vi "UHR-Fleezers Control (host) - 10.8.vi"() -> ()   [LabVIEW 2013] (continued)
            n877 = local read "Pump write delay (ms)"() -> (w1433:dbl)
            n878 = flat-sequence {
              tunnel: w1432 -> [w1446]
              tunnel: w1433 -> [w1442]
              tunnel: w1431 -> [_]
              tunnel: w1433 -> [w1448]
              tunnel: w1432 -> [w1449]
              frame #0 {
                n879 = local read "All Pump Parameters"() -> (w1441:T5)
                n880 = Multiply(x=60.0, y="Flush Center Ch Rate (ul/m)") -> (x*y=w1438:dbl)
                n881 = Unbundle By Name(w1441) -> ("Pump 2"=w1447:T35)
                n882 = call "Set pump parameters.vi"("Pump write delay (ms)"=w1442, "Volume (uL)"="Flush Center Ch Volume (uL)", "Rate (uL/h)"=w1438, "Units"=3.0, "Pump #"=2.0, "Pump Parameters In"=w1447, "VISA resource name"=w1446) -> ("Pump Parameters Out"=w1440:T35)  [unwired: 3 in]
                n883 = Bundle By Name(cluster=w1441, "Pump 2"=w1440) -> (w1439:T5)
                n884 = local write "All Pump Parameters"(w1439) -> ()
                n885 = Add(x="Flush Center Ch Volume (uL)", y="Total Volume\nFlushed (uL)") -> (x+y=w1435:dbl)
                n886 = local write "Total Volume\nFlushed (uL)"(w1435) -> ()
              }
              frame #1 {
                n887 = Wait (ms)(milliseconds to wait=w1448) -> ()  [unwired: 1 out]
              }
              frame #2 {
                n888 = call "Write to pump.vi"("string"="start", "VISA resource name"=w1449) -> ()  [unwired: 1 out]
              }
            }
            n889 = local read "Chemyx Syringe Pump Serial Port"() -> (w1432:refnum<visa-resource-name>)
          }
          frame Enabled {
            n890 = call "hamilton_controller.vi"("Open?"=w1451, "valve"=enum16{"A", "B", "C", "D", "ALL"}."B", "action"=T21."MOVE VALVE") -> ()  [unwired: 8 in, 1 out]
          }
        }
      }
      event "Sample Channel Flow": Value Change {
        n891 = event-data() -> ()  [unwired: 7 out]
        n892 = call "hamilton_controller.vi"("Open?"="Sample Channel Flow", "valve"=enum16{"A", "B", "C", "D", "ALL"}."C", "action"=T21."MOVE VALVE") -> ()  [unwired: 8 in, 1 out]
      }
      event "Flip Green Filter": Value Change {
        n893 = event-data() -> ()  [unwired: 7 out]
        n894 = Not(x="Flip Green Filter") -> (.not. x?=w1457:bool)
        n895 = local write "Flip Green Filter"(w1457) -> ()
        n896 = flat-sequence {
          tunnel: w1465 -> [w1470]
          tunnel: w1464 -> [w1469]
          tunnel: [w1467] -> w1462
          tunnel: [w1466] -> w1461
          tunnel: [w1472] -> w1460
          tunnel: w1462 -> [w1472]
          tunnel: [w1471] -> w1459
          tunnel: w1461 -> [w1471]
          tunnel: w1460 -> [w1476]
          tunnel: w1459 -> [w1475]
          tunnel: [w1474] -> w1463
          frame #0 {
            n897 = xnode "Read/Write Control"("FPGA VI Reference In"=w1470, "error in"=w1469, "Green Filter Flipper"=TRUE) -> ("FPGA VI Reference Out"=w1467:T19, "error out"=w1466:errorcluster)
          }
          frame #1 {
            n898 = Wait (ms)(milliseconds to wait=u32 100) -> ()  [unwired: 1 out]
          }
          frame #2 {
            n899 = xnode "Read/Write Control"("FPGA VI Reference In"=w1476, "error in"=w1475, "Green Filter Flipper"=FALSE) -> ("error out"=w1474:errorcluster)  [unwired: 1 out]
          }
        }
      }
      event "Pump 1 contents", "Pump 3 contents": Value Change {
        n900 = event-data() -> ()  [unwired: 7 out]
        n901 = local read "Pump 1 contents"() -> (→"Pump 1 cont disp":string)
        n902 = local read "Pump 3 contents"() -> (→"Pump 3 cont disp":string)
      }
      event "Reset Trap Pos. FB": Value Change {
        n903 = event-data() -> ()  [unwired: 7 out]
        n904 = xnode "Read/Write Control"("FPGA VI Reference In"=w1482, "error in"=w1481, "Trap Pos. FB Reset"="Reset Trap Pos. FB") -> ()  [unwired: 2 out]
      }
      event "Trap Pos. FB ON": Value Change {
        n905 = event-data() -> ()  [unwired: 7 out]
        n906 = xnode "Read/Write Control"("FPGA VI Reference In"=w1485, "error in"=w1484, "Force feedback"="Trap Pos. FB ON") -> ()  [unwired: 2 out]
      }
      event "Trap Pos. FB Range", "Trap Pos. FB Gains", "Trap Pos. FB Mult Factor", "Trap Pos. FB Offset Factor", "Trap Pos FB Negate Action", "Trap Pos FB Monitor\nT1 or T2": Value Change {
        n907 = event-data() -> ()  [unwired: 7 out]
        n908 = xnode "Read/Write Control"("FPGA VI Reference In"=w1494, "error in"=w1493, "Trap Pos. FB Range"="Trap Pos. FB Range", "Trap Pos. FB Gains"="Trap Pos. FB Gains", "Trap Pos. FB Mult Factor"="Trap Pos. FB Mult Factor", "Trap Pos. FB Offset Factor"="Trap Pos. FB Offset Factor", "Trap Pos FB Negate Action"="Trap Pos FB Negate Action", "Trap Pos FB Monitor T1 or T2"="Trap Pos FB Monitor\nT1 or T2", "AI1 X Scale"="Trap Pos. AI1 X Pre-scale") -> ()  [unwired: 2 out]
      }
      event "Trap Pos FB SP": Value Change {
        n909 = event-data() -> ()  [unwired: 7 out]
        n910 = xnode "Read/Write Control"("FPGA VI Reference In"=w1497, "error in"=w1496, "Trap Pos. FB SP"="Trap Pos FB SP") -> ()  [unwired: 2 out]
      }
      event "Set SP to Reading": Value Change {
        n911 = event-data() -> ()  [unwired: 7 out]
        n912 = local read "Trap Pos FB Monitor\nT1 or T2"() -> (w1505:bool)
        n913 = local read "Trap X AI1 (DMA)"() -> (w1508:T13)
        n914 = local read "Trap X (AI1)"() -> (w1511:T10)
        n915 = Unbundle By Name(w1511) -> ("Trap 1"=w1510:fxp<+/-,16,1>, "Trap 2"=w1509:fxp<+/-,16,1>)
        n916 = Unbundle By Name(w1508) -> ("Set 1"=w1507:fxp<+/-,16,1>, "Set 2"=w1506:fxp<+/-,16,1>)
        n917 = Select(t=w1510, s=w1505, f=w1509) -> (s? t:f=w1504:fxp<+/-,16,1>)
        n918 = Select(t=w1507, s=w1505, f=w1506) -> (s? t:f=w1503:fxp<+/-,16,1>)
        n919 = Not(x="Set SP Using...") -> (.not. x?=w1498:bool)
        n920 = Select(t=w1504, s=w1498, f=w1503) -> (s? t:f=w1499:fxp<+/-,16,1>)
        n921 = xnode "Read/Write Control"("FPGA VI Reference In"=w1501, "error in"=w1500, "Trap Pos. FB SP"=w1499) -> ()  [unwired: 2 out]
        n922 = local write "Trap Pos FB SP"(w1499) -> ()
      }
      event "Trap Pos. FB Out Scale 2^n": Value Change {
        n923 = event-data() -> ()  [unwired: 7 out]
        n924 = Scale By Power Of 2(n="Trap Pos. FB Out Scale 2^n", x=ext 1.0) -> (x*2^n=w1513:ext)
        n925 = property on="Trap Pos. FB Mult Factor" class="DigNum (strict)"("Val(Sgnl)"=w1513) -> ()  [unwired: 2 in, 2 out]
      }
      event "Trap Pos FB Int Count": Value Change {
        n926 = event-data() -> ()  [unwired: 7 out]
        n927 = xnode "Read/Write Control"("FPGA VI Reference In"=w1518, "error in"=w1517, "Trap Pos FB Int Count"="Trap Pos FB Int Count") -> ()  [unwired: 2 out]
      }
    }
    "error out 2" <- w637
    n928 = node-c288() -> ()  [unwired: 1 in, 1 out]
  }
  n929 = timed-loop "Run Scripts, including: stage motion" {
    timing: w68 -> [_]
    timing-out: [_] -> w67
    tunnel: w16 -> [_]
    stop <- w1520 stop-if-true
    n930 = node-c288() -> ()  [unwired: 1 in, 1 out]
    n931 = event shown="[10] \"Move to Position 1\", \"Move to Position 2\", \"Move to Position 3\", \"Move to Position 4\", \"Move to Position 5\", \"Lower Ch. Cap.\": Value Change" {
      selector: _ -> [_ _ _ _ _ _ _ _ _ _ _ _ _ _ _ _ _]
      dyn-events: _ -> [_ _ _ _ _ _ _ _ _ _ _ _ _ _ _ _ _]
      timeout: 50 -> [_ _ _ _ _ _ _ _ _ _ _ _ _ _ _ _ _]
      tunnel: ["Set Position" "Move to Position" "Move Cap. 1 (DNA Top)" _ "Move Cap. 2 (ADig Bot)" _ "Cal/Data Acq. Spot" "Dump Beads" "Dip for Protein" _ _ "Got ADig bead" "Got DNA bead" "Take Stepping Data" _ "Take Detection Laser\nImage" _] -> _
      tunnel: [_ _ _ _ _ _ _ _ _ _ _ _ _ _ _ _ w1905] -> w1520
      event "Set Position", "Set Position 2", "Set Position 3", "Set Position 4", "Set Position 5", "Set Position 1": Value Change {
        n932 = event-data() -> ()  [unwired: 1 in, 5 out]
        n933 = Build Array("Set Position 1", "Set Position 2", "Set Position 3", "Set Position 4", "Set Position 5") -> (w1539:bool[])
        n934 = Boolean Array To Number(Boolean array=w1539) -> (number=w1538:u32)
        n935 = Logarithm Base 2(1:w1538) -> (0:w1530:dbl)
        n936 = call "CONEX_FUNCTIONAL_GLOBAL.vi"("Command"=T20."GET POS") -> ("Current Position"=w1523:dbl[])  [unwired: 8 in, 2 out]
        n937 = Decrement(x="Position") -> (x-1=w1528:dbl)
        n938 = Greater Or Equal?(x=w1530, y=0.0) -> (x >= y?=w1531:bool)
        n939 = Select(t=w1530, s=w1531, f=w1528) -> (s? t:f=w1527:dbl)
        n940 = Increment(x=w1527) -> (x+1=w1526:dbl)
        n941 = Build Array (concatenate)(w1526, w1523) -> (w1525:dbl[])
        n942 = Replace Array Subset(array="Saved Stage Positions", new element=w1525, index (row)=w1527) -> (w1540:dbl[][])  [unwired: 1 in]
        n943 = local write "Saved Stage Positions"(w1540) -> ()
      }
      event "Move to Position": Value Change {
        n944 = event-data() -> ()  [unwired: 1 in, 5 out]
        n945 = flat-sequence {
          frame #0 {
            n946 = local read "Position"() -> (w1555:dbl)
            n947 = local read "Saved Stage Positions"() -> (w1553:dbl[][])
            n948 = Decrement(x=w1555) -> (x-1=w1552:dbl)
            n949 = Array Subset(array=w1553, index (row)=w1552, length (row)=1 ("length"), index (col)=1 ("index"), length (col)=3 ("length")) -> (w1549:dbl[][])
            n950 = Reshape Array(w1549, 3 ("dimension size")) -> (w1545:dbl[])
            n951 = local write "Stage Moving"(TRUE ("Stage Moving")) -> ()
            n952 = call "CONEX_FUNCTIONAL_GLOBAL.vi"("Axis"=enum16{"X", "Y", "Z", "XY", "XZ", "YZ", "XYZ"}."XYZ", "Position"=w1545, "Command"=T20."ABS MOVE") -> ()  [unwired: 6 in, 3 out]
          }
          frame #1 {
            n953 = call "motor_done_moving.vi"("wait at least (s)"=0.0) -> ()  [unwired: 11 in]
          }
          frame #2 {
            n954 = call <vilib>:"Beep.vi"() -> ()  [unwired: 3 in, 9 out]
            n955 = local write "Stage Moving"(FALSE ("Stage Moving")) -> ()
          }
        }
      }
      event "Move Cap. 1 (DNA Top)": Value Change {
        n956 = event-data() -> ()  [unwired: 1 in, 5 out]
        n957 = local write "Move Cap. 1 (DNA Top)"(FALSE ("Move Cap. 1 (DNA Right)")) -> ()
        n958 = flat-sequence {
          tunnel: ["Cap 1 Samp Flow ON"] -> w1559
          tunnel: w1559 -> [w1578]
          tunnel: [w1578] -> w1558
          tunnel: w1558 -> [w1579]
          frame #0 {
            n959 = local read "Saved Stage Positions"() -> (w1572:dbl[][])
            n960 = Array Subset(array=w1572, index (row)=0 ("index"), length (row)=1 ("length"), index (col)=1 ("index"), length (col)=3 ("length")) -> (w1569:dbl[][])
            n961 = Reshape Array(w1569, 3 ("dimension size")) -> (w1563:dbl[])
            n962 = case "start flow in central channel to wash" shown="True" "Cap 1 Samp Flow ON" {
              frame False {
              }
              frame True {
                n963 = call "hamilton_controller.vi"("Open?"=TRUE, "valve"=enum16{"A", "B", "C", "D", "ALL"}."C", "action"=T21."MOVE VALVE") -> ()  [unwired: 8 in, 1 out]
              }
            }
            n964 = call "CONEX_FUNCTIONAL_GLOBAL.vi"("Axis"=enum16{"X", "Y", "Z", "XY", "XZ", "YZ", "XYZ"}."XYZ", "Position"=w1563, "Command"=T20."ABS MOVE") -> ()  [unwired: 6 in, 3 out]
            n965 = local write "Stage Moving"(TRUE ("Stage Moving")) -> ()
          }
          frame #1 {
            n966 = call "motor_done_moving.vi"("wait at least (s)"=2.0) -> ()  [unwired: 11 in]
          }
          frame #2 {
            n967 = local write "Stage Moving"(FALSE ("Stage Moving")) -> ()
            n968 = case "stop flow" shown="True" w1579 {
              frame False {
              }
              frame True {
                n969 = call "hamilton_controller.vi"("Open?"=FALSE, "valve"=enum16{"A", "B", "C", "D", "ALL"}."C", "action"=T21."MOVE VALVE") -> ()  [unwired: 8 in, 1 out]
              }
            }
            n970 = case shown="True" TRUE {
              tunnel: "Cap 1 T ON" -> [w1588 w1589]
              frame False {
                n971 = property on="Trap 1 (ON/OFF)" class="Bool (strict)"("Val(Sgnl)"=w1588) -> ()  [unwired: 2 in, 2 out]
              }
              frame True {
                n972 = property on="Trap 2 (ON/OFF)" class="Bool (strict)"("Val(Sgnl)"=w1589) -> ()  [unwired: 2 in, 2 out]
              }
            }
            n973 = call <vilib>:"Beep.vi"() -> ()  [unwired: 3 in, 9 out]
            n974 = case shown="True" "Cap 1 Flow ON" {
              frame False {
              }
              frame True {
                n975 = property on="Inject Top" class="Bool (strict)"("Val(Sgnl)"=TRUE ("Value (Signaling)")) -> ()  [unwired: 2 in, 2 out]
              }
            }
          }
        }
      }
      event Timeout {
        n976 = event-data() -> ()  [unwired: 1 in, 2 out]
      }
      event "Move Cap. 2 (ADig Bot)": Value Change {
        n977 = event-data() -> ()  [unwired: 1 in, 5 out]
        n978 = local write "Move Cap. 2 (ADig Bot)"(FALSE ("Move Cap. 2 (ADig Left)")) -> ()
        n979 = flat-sequence {
          tunnel: ["Cap 2 Samp Flow ON"] -> w1591
          tunnel: w1591 -> [w1610]
          tunnel: [w1610] -> w1590
          tunnel: w1590 -> [w1611]
          frame #0 {
            n980 = local read "Saved Stage Positions"() -> (w1604:dbl[][])
            n981 = case shown="True" "Cap 2 Samp Flow ON" {
              frame False {
              }
              frame True {
                n982 = call "hamilton_controller.vi"("Open?"=TRUE, "valve"=enum16{"A", "B", "C", "D", "ALL"}."C", "action"=T21."MOVE VALVE") -> ()  [unwired: 8 in, 1 out]
              }
            }
            n983 = Array Subset(array=w1604, index (row)=1 ("index"), length (row)=1 ("length"), index (col)=1 ("index"), length (col)=3 ("length")) -> (w1601:dbl[][])
            n984 = Reshape Array(w1601, 3 ("dimension size")) -> (w1595:dbl[])
            n985 = local write "Stage Moving"(TRUE ("Stage Moving")) -> ()
            n986 = call "CONEX_FUNCTIONAL_GLOBAL.vi"("Axis"=enum16{"X", "Y", "Z", "XY", "XZ", "YZ", "XYZ"}."XYZ", "Position"=w1595, "Command"=T20."ABS MOVE") -> ()  [unwired: 6 in, 3 out]
          }
          frame #1 {
            n987 = call "motor_done_moving.vi"("wait at least (s)"=2.0) -> ()  [unwired: 11 in]
          }
          frame #2 {
            n988 = local write "Stage Moving"(FALSE ("Stage Moving")) -> ()
            n989 = case shown="True" TRUE {
              tunnel: "Cap 2 T ON" -> [w1620 w1621]
              frame False {
                n990 = property on="Trap 2 (ON/OFF)" class="Bool (strict)"("Val(Sgnl)"=w1620) -> ()  [unwired: 2 in, 2 out]
              }
              frame True {
                n991 = property on="Trap 1 (ON/OFF)" class="Bool (strict)"("Val(Sgnl)"=w1621) -> ()  [unwired: 2 in, 2 out]
              }
            }
            n992 = call <vilib>:"Beep.vi"() -> ()  [unwired: 3 in, 9 out]
            n993 = case shown="True" w1611 {
              frame False {
              }
              frame True {
                n994 = call "hamilton_controller.vi"("Open?"=FALSE, "valve"=enum16{"A", "B", "C", "D", "ALL"}."C", "action"=T21."MOVE VALVE") -> ()  [unwired: 8 in, 1 out]
              }
            }
            n995 = case shown="True" "Cap 2 Flow ON" {
              frame False {
              }
              frame True {
                n996 = property on="Inject Bottom" class="Bool (strict)"("Val(Sgnl)"=TRUE ("Value (Signaling)")) -> ()  [unwired: 2 in, 2 out]
              }
            }
          }
        }
      }
      event "+z", "-z": Value Change {
        n997 = event-data() -> ()  [unwired: 1 in, 5 out]
        n998 = flat-sequence {
          frame #0 {
            w1623 = 0.0 ("element")
            n999 = Divide(x="z nudge increment (um)", y=1000.0) -> (x/y=w1636:dbl)
            n1000 = Boolean To (0,1)(Boolean="+z") -> (0, 1=w1629:i16)
            n1001 = Boolean To (0,1)(Boolean="-z") -> (0, 1=w1630:i16)
            n1002 = Multiply(x=w1629, y=w1636) -> (x*y=w1633:dbl)
            n1003 = Multiply(x=w1630, y=w1636) -> (x*y=w1631:dbl)
            n1004 = Negate(x=w1631) -> (-x=w1632:dbl)
            n1005 = Add(x=w1633, y=w1632) -> (x+y=w1624:dbl)
            n1006 = Build Array(w1623, w1623, w1624) -> (w1622:dbl[])
            n1007 = call "CONEX_FUNCTIONAL_GLOBAL.vi"("Axis"=enum16{"X", "Y", "Z", "XY", "XZ", "YZ", "XYZ"}."Z", "Position"=w1622, "Command"=T20."REL MOVE") -> ()  [unwired: 6 in, 3 out]
            n1008 = local write "Stage Moving"(TRUE ("Stage Moving")) -> ()
          }
          frame #1 {
            n1009 = local write "Stage Moving"(FALSE ("Stage Moving")) -> ()
            n1010 = call <vilib>:"Beep.vi"() -> ()  [unwired: 3 in, 9 out]
          }
        }
      }
      event "Cal/Data Acq. Spot": Value Change {
        # "wait for calibration file\nto be written"
        # "signal save cal true\nthis tells the data \nacquisition loop to\nstart sending the data\nto a calibration file"
        # "separate traps to\nthe desired trap delta"
        # "move stage to data acquisition spot"
        # "CHANGE FISH FOR TETHER BACK\nTO TRUE VALUE HERE."
        n1011 = event-data() -> ()  [unwired: 1 in, 5 out]
        n1012 = local write "Cal/Data Acq. Spot"(FALSE ("Cal/Data Acq. Spot")) -> ()
        n1013 = flat-sequence {
          tunnel: ["Cal @ (MHz)"] -> w1639
          tunnel: w1639 -> [w1662]
          tunnel: w1639 -> [w1683]
          frame #0 {
            n1014 = local read "Saved Stage Positions"() -> (w1647:dbl[][])
            n1015 = Array Subset(array=w1647, index (row)=2 ("index"), length (row)=1 ("length"), index (col)=1 ("index"), length (col)=3 ("length")) -> (w1650:dbl[][])
            n1016 = Reshape Array(w1650, 3 ("dimension size")) -> (w1643:dbl[])
            n1017 = local write "Stage Moving"(TRUE ("Stage Moving")) -> ()
            n1018 = call "CONEX_FUNCTIONAL_GLOBAL.vi"("Axis"=enum16{"X", "Y", "Z", "XY", "XZ", "YZ", "XYZ"}."XYZ", "Position"=w1643, "Command"=T20."ABS MOVE") -> ()  [unwired: 6 in, 3 out]
          }
          frame #1 {
            n1019 = call "motor_done_moving.vi"("wait at least (s)"=2.0) -> ()  [unwired: 11 in]
          }
          frame #2 {
            n1020 = property on="Trap Delta (MHz)" class="DigNum (strict)"("Val(Sgnl)"="Cal @ (MHz)") -> ()  [unwired: 2 in, 2 out]
            n1021 = local write "Stage Moving"(FALSE ("Stage Moving")) -> ()
            n1022 = call <vilib>:"Beep.vi"() -> ()  [unwired: 3 in, 9 out]
          }
          frame #3 {
            n1023 = Wait (ms)(milliseconds to wait=u32 100) -> ()  [unwired: 1 out]
          }
          frame #4 {
            n1024 = property on="Save Calibration" class="Bool (strict)"("Val(Sgnl)"=TRUE ("Value (Signaling)")) -> ()  [unwired: 2 in, 2 out]
          }
          frame #5 {
            n1025 = Wait (ms)(milliseconds to wait=u32 4000) -> ()  [unwired: 1 out]
          }
          frame #6 {
            n1026 = while {
              stop <- w1659 stop-if-true
              n1027 = local read "Saving..."() -> (w1660:bool)
              n1028 = Wait (ms)(milliseconds to wait=u32 100) -> ()  [unwired: 1 out]
              n1029 = Not(x=w1660) -> (.not. x?=w1659:bool)
            }
          }
          frame #7 {
            n1030 = case shown="True" "W/ Offset 1" {
              tunnel: w1662 -> [_ w1664]
              frame False {
              }
              frame True {
                n1031 = stacked-sequence {
                  tunnel: w1664 -> [_ _ _ _ _ _ _ w1681]
                  frame #0 {
                    n1032 = Replace Array Subset(array=u32[] [0] ("Index Values"), new element="Offset 1 Set", index=0) -> (w1665:u32[])
                    n1033 = property on="Saved AOD Raster Scan Parameter Sets" class="Arr (strict)"("Index Values"=w1665) -> ()  [unwired: 2 in, 2 out]
                    n1034 = property on="Trap Delta (MHz)" class="DigNum (strict)"("Val(Sgnl)"="Offset 1 Start (MHz)") -> ()  [unwired: 2 in, 2 out]
                  }
                  frame #1 {
                    n1035 = Wait (ms)(milliseconds to wait=u32 200) -> ()  [unwired: 1 out]
                  }
                  frame #2 {
                    n1036 = property on="Load parameters" class="Bool (strict)"("Val(Sgnl)"=TRUE ("Value (Signaling)")) -> ()  [unwired: 2 in, 2 out]
                  }
                  frame #3 {
                    n1037 = Wait (ms)(milliseconds to wait=u32 200) -> ()  [unwired: 1 out]
                  }
                  frame #4 {
                    n1038 = property on="Trap Raster Scan" class="Bool (strict)"("Val(Sgnl)"=TRUE ("Value (Signaling)")) -> ()  [unwired: 2 in, 2 out]
                  }
                  frame #5 {
                    n1039 = Wait (ms)(milliseconds to wait=u32 2000) -> ()  [unwired: 1 out]
                  }
                  frame #6 {
                    n1040 = while {
                      stop <- w1678 stop-if-true
                      n1041 = local read "Raster Scanning..."() -> (w1680:bool)
                      n1042 = local read "Saving..."() -> (w1676:bool)
                      n1043 = Wait (ms)(milliseconds to wait=u32 100) -> ()  [unwired: 1 out]
                      n1044 = Not(x=w1676) -> (.not. x?=w1675:bool)
                      n1045 = Not(x=w1680) -> (.not. x?=w1677:bool)
                      n1046 = And(x=w1677, y=w1675) -> (x .and. y?=w1678:bool)
                    }
                  }
                  frame #7 {
                    n1047 = property on="Trap Delta (MHz)" class="DigNum (strict)"("Val(Sgnl)"=w1681) -> ()  [unwired: 2 in, 2 out]
                  }
                }
              }
            }
          }
          frame #8 {
            n1048 = local read "Save ave N"() -> (w1682:dbl)
            n1049 = case shown="True" "W/ Offset 2" {
              tunnel: w1683 -> [_ w1689]
              tunnel: w1682 -> [_ w1688]
              frame False {
                n1050 = Multiply(x="Cal read wait (s)", y=u32 1000 ("milliseconds to wait")) -> (x*y=w1686:u32)
                n1051 = Wait (ms)(milliseconds to wait=w1686) -> ()  [unwired: 1 out]
              }
              frame True {
                n1052 = stacked-sequence {
                  tunnel: w1689 -> [_ _ _ _ _ _ _ _ _ w1710 _ _]
                  tunnel: w1688 -> [_ _ _ _ _ _ _ _ _ w1708 _ _]
                  frame #0 {
                    n1053 = property on="Save ave N" class="DigNum (strict)"("Val(Sgnl)"=1.0 ("Value (Signaling)")) -> ()  [unwired: 2 in, 2 out]
                  }
                  frame #1 {
                    n1054 = Wait (ms)(milliseconds to wait=u32 500) -> ()  [unwired: 1 out]
                  }
                  frame #2 {
                    n1055 = property on="Trap Delta (MHz)" class="DigNum (strict)"("Val(Sgnl)"="Offset 2 Start (MHz)") -> ()  [unwired: 2 in, 2 out]
                    n1056 = Replace Array Subset(array=u32[] [0] ("Index Values"), new element="Offset 2 Set", index=0) -> (w1694:u32[])
                    n1057 = property on="Saved AOD Raster Scan Parameter Sets" class="Arr (strict)"("Index Values"=w1694) -> ()  [unwired: 2 in, 2 out]
                  }
                  frame #3 {
                    n1058 = Wait (ms)(milliseconds to wait=u32 500) -> ()  [unwired: 1 out]
                  }
                  frame #4 {
                    n1059 = property on="Load parameters" class="Bool (strict)"("Val(Sgnl)"=TRUE ("Value (Signaling)")) -> ()  [unwired: 2 in, 2 out]
                  }
                  frame #5 {
                    n1060 = Wait (ms)(milliseconds to wait=u32 500) -> ()  [unwired: 1 out]
                  }
                  frame #6 {
                    n1061 = property on="Trap Raster Scan" class="Bool (strict)"("Val(Sgnl)"=TRUE ("Value (Signaling)")) -> ()  [unwired: 2 in, 2 out]
                  }
                  frame #7 {
                    n1062 = Wait (ms)(milliseconds to wait=u32 2000) -> ()  [unwired: 1 out]
                  }
                  frame #8 {
                    n1063 = while {
                      stop <- w1703 stop-if-true
                      n1064 = local read "Raster Scanning..."() -> (w1706:bool)
                      n1065 = local read "Saving..."() -> (w1704:bool)
                      n1066 = Wait (ms)(milliseconds to wait=u32 100) -> ()  [unwired: 1 out]
                      n1067 = Not(x=w1704) -> (.not. x?=w1702:bool)
                      n1068 = Not(x=w1706) -> (.not. x?=w1705:bool)
                      n1069 = And(x=w1705, y=w1702) -> (x .and. y?=w1703:bool)
                    }
                  }
                  frame #9 {
                    n1070 = property on="Trap Delta (MHz)" class="DigNum (strict)"("Val(Sgnl)"=w1710) -> ()  [unwired: 2 in, 2 out]
                    n1071 = property on="Saved AOD Raster Scan Parameter Sets" class="Arr (strict)"("Index Values"=u32[] [0]) -> ()  [unwired: 2 in, 2 out]
                    n1072 = property on="Save ave N" class="DigNum (strict)"("Val(Sgnl)"=w1708) -> ()  [unwired: 2 in, 2 out]
                  }
                  frame #10 {
                    n1073 = Wait (ms)(milliseconds to wait=u32 500) -> ()  [unwired: 1 out]
                  }
                  frame #11 {
                    n1074 = property on="Load parameters" class="Bool (strict)"("Val(Sgnl)"=TRUE ("Value (Signaling)")) -> ()  [unwired: 2 in, 2 out]
                  }
                }
              }
            }
          }
          frame #9 {
            n1075 = property on="Read Cal" class="Bool (strict)"("Val(Sgnl)"=TRUE ("Value (Signaling)")) -> ()  [unwired: 2 in, 2 out]
          }
          frame #10 {
            n1076 = Wait (ms)(milliseconds to wait=u32 500) -> ()  [unwired: 1 out]
          }
          frame #11 {
            n1077 = property on="Fish for Tether" class="Bool (strict)"("Val(Sgnl)"=TRUE ("Value (Signaling)")) -> ()  [unwired: 2 in, 2 out]
          }
        }
      }
      event "Dump Beads": Value Change {
        # "SCRIPT TO REMOVE BOTH BEADS FROM THE TRAPS. TURNS ON LIGHT WHICH INDICATES THAT STAGE IS MOVING. THEN STOPS SAVING DATA. \nSETS Sample Channel Flow TO TRUE. STOPS INTERLACING GREEN FLUORESCENCE. TURNS OFF Tether INDICATOR BECAUSE WE ARE THROWING IT\nAWAY. SHUTS OFF TRAP POSITION FEEDBACK."
        n1078 = event-data() -> ()  [unwired: 1 in, 5 out]
        n1079 = flat-sequence {
          frame #0 {
            w1717 = FALSE ("Fl. Triggered...")
            w1718 = TRUE ("Stage Moving")
            n1080 = local read "Saving..."() -> (w1719:bool)
            n1081 = local write "Fl. Triggered..."(w1717) -> ()
            n1082 = local write "Stage Moving"(w1718) -> ()
            n1083 = local write "Tether"(w1717) -> ()
            n1084 = property on="Green Laser ON/Interlacing" class="Bool (strict)"("Val(Sgnl)"=w1717) -> ()  [unwired: 2 in, 2 out]
            n1085 = property on="Trap Pos. FB ON" class="Bool (strict)"("Val(Sgnl)"=w1717) -> ()  [unwired: 2 in, 2 out]
            n1086 = property on="Sample Channel Flow" class="Bool (strict)"("Val(Sgnl)"=w1718) -> ()  [unwired: 2 in, 2 out]
            n1087 = local write "Stop Saving"(w1719) -> ()
          }
          frame #1 {
            # "MOVES TO THE DUMP BEADS POSITION"
            n1088 = local read "Saved Stage Positions"() -> (w1723:dbl[][])
            n1089 = Array Subset(array=w1723, index (row)=3 ("index"), length (row)=1 ("length"), index (col)=1 ("index"), length (col)=3 ("length")) -> (w1726:dbl[][])
            n1090 = Reshape Array(w1726, 3 ("dimension size")) -> (w1721:dbl[])
            n1091 = call "CONEX_FUNCTIONAL_GLOBAL.vi"("Axis"=enum16{"X", "Y", "Z", "XY", "XZ", "YZ", "XYZ"}."XYZ", "Position"=w1721, "Command"=T20."ABS MOVE") -> ()  [unwired: 6 in, 3 out]
          }
          frame #2 {
            n1092 = call "motor_done_moving.vi"("wait at least (s)"=2.0) -> ()  [unwired: 11 in]
          }
          frame #3 {
            w1731 = FALSE ("Value (Signaling)")
            # "TURNS TRAPS OFF SO THAT\nBEADS REMAIN AT DUMP \nBEADS POSITION"
            n1093 = property on="Trap 1 (ON/OFF)" class="Bool (strict)"("Val(Sgnl)"=w1731) -> ()  [unwired: 2 in, 2 out]
            n1094 = property on="Trap 2 (ON/OFF)" class="Bool (strict)"("Val(Sgnl)"=w1731) -> ()  [unwired: 2 in, 2 out]
            n1095 = call <vilib>:"Beep.vi"() -> ()  [unwired: 3 in, 9 out]
          }
          frame #4 {
            n1096 = local read "Cal @ (MHz)"() -> (w1732:dbl)
            n1097 = property on="Trap Delta (MHz)" class="DigNum (strict)"("Val(Sgnl)"=w1732) -> ()  [unwired: 2 in, 2 out]
          }
          frame #5 {
            # "MOVES STAGE BACK TO THE\nANTIDIG CAPILARY BY CALLING\nTHE Move Cap. 2 SCRIPT"
            n1098 = property on="Move Cap. 2 (ADig Bot)" class="Bool (strict)"("Val(Sgnl)"=TRUE ("Value (Signaling)")) -> ()  [unwired: 2 in, 2 out]
          }
        }
      }
      event "Dip for Protein": Value Change {
        n1099 = event-data() -> ()  [unwired: 1 in, 5 out]
        n1100 = flat-sequence {
          frame #0 {
            n1101 = case shown="True" "Move Trap Before?" {
              frame False {
              }
              frame True {
                n1102 = property on="Trap Delta (MHz)" class="DigNum (strict)"("Val(Sgnl)"="Dip Trap Delta 1 (MHz)") -> ()  [unwired: 2 in, 2 out]
              }
            }
          }
          frame #1 {
            n1103 = local read "Saved Stage Positions"() -> (w1740:dbl[][])
            n1104 = Array Subset(array=w1740, index (row)=4 ("index"), length (row)=1 ("length"), index (col)=1 ("index"), length (col)=3 ("length")) -> (w1743:dbl[][])
            n1105 = Reshape Array(w1743, 3 ("dimension size")) -> (w1738:dbl[])
            n1106 = call "CONEX_FUNCTIONAL_GLOBAL.vi"("Axis"=enum16{"X", "Y", "Z", "XY", "XZ", "YZ", "XYZ"}."XYZ", "Position"=w1738, "Command"=T20."ABS MOVE") -> ()  [unwired: 6 in, 3 out]
          }
          frame #2 {
            n1107 = Multiply(x="Duration (s)", y=1000.0) -> (x*y=w1747:dbl)
            n1108 = Wait (ms)(milliseconds to wait=w1747) -> ()  [unwired: 1 out]
          }
          frame #3 {
            n1109 = local read "Saved Stage Positions"() -> (w1753:dbl[][])
            n1110 = Array Subset(array=w1753, index (row)=2 ("index"), length (row)=1 ("length"), index (col)=1 ("index"), length (col)=3 ("length")) -> (w1756:dbl[][])
            n1111 = Reshape Array(w1756, 3 ("dimension size")) -> (w1751:dbl[])
            n1112 = call "CONEX_FUNCTIONAL_GLOBAL.vi"("Axis"=enum16{"X", "Y", "Z", "XY", "XZ", "YZ", "XYZ"}."XYZ", "Position"=w1751, "Command"=T20."ABS MOVE") -> ()  [unwired: 6 in, 3 out]
          }
          frame #4 {
            n1113 = case shown="True" "Move Trap After?" {
              frame False {
              }
              frame True {
                n1114 = property on="Trap Delta (MHz)" class="DigNum (strict)"("Val(Sgnl)"="Dip Trap Delta 2 (MHz)") -> ()  [unwired: 2 in, 2 out]
              }
            }
          }
          frame #5 {
            n1115 = case shown="True" "Green ON After?" {
              frame False {
              }
              frame True {
                n1116 = property on="Green Laser ON/Interlacing" class="Bool (strict)"("Val(Sgnl)"=TRUE ("Value (Signaling)")) -> ()  [unwired: 2 in, 2 out]
              }
            }
          }
          frame #6 {
            n1117 = Wait (ms)(milliseconds to wait=u32 500) -> ()  [unwired: 1 out]
          }
          frame #7 {
            n1118 = case shown="True" "Save Data After?" {
              frame False {
              }
              frame True {
                n1119 = property on="Start Saving" class="Bool (strict)"("Val(Sgnl)"=TRUE ("Value (Signaling)")) -> ()  [unwired: 2 in, 2 out]
              }
            }
          }
        }
      }
      event "Profile": Value Change {
        n1120 = event-data() -> ()  [unwired: 1 in, 5 out]
        n1121 = flat-sequence {
          tunnel: [w1769] -> w1768
          tunnel: w1768 -> [w1773]
          tunnel: [w1772] -> w1767
          tunnel: w1767 -> [w1779]
          frame #0 {
            w1770 = 0.0 ("element")
            n1122 = Build Array(w1770, "Y change (mm)", w1770) -> (w1769:dbl[])
          }
          frame #1 {
            # "move to new position and start saving"
            n1123 = local write "Stage Moving"(TRUE ("Stage Moving")) -> ()
            n1124 = local write "Start Saving"(TRUE ("Start Saving")) -> ()
            n1125 = call "CONEX_FUNCTIONAL_GLOBAL.vi"("Axis"=enum16{"X", "Y", "Z", "XY", "XZ", "YZ", "XYZ"}."Y", "Position"=w1773, "Command"=T20."REL MOVE") -> ()  [unwired: 6 in, 3 out]
            n1126 = Negate(x=w1773) -> (-x=w1772:dbl[])
          }
          frame #2 {
            # "go back to start"
            n1127 = call "CONEX_FUNCTIONAL_GLOBAL.vi"("Axis"=enum16{"X", "Y", "Z", "XY", "XZ", "YZ", "XYZ"}."Y", "Position"=w1779, "Command"=T20."REL MOVE") -> ()  [unwired: 6 in, 3 out]
          }
          frame #3 {
            # "stop saving"
            n1128 = local write "Stop Saving"(TRUE ("Stop Saving")) -> ()
            n1129 = local write "Stage Moving"(FALSE ("Stage Moving")) -> ()
          }
        }
      }
      event "Move to Position 1", "Move to Position 2", "Move to Position 3", "Move to Position 4", "Move to Position 5", "Lower Ch. Cap.": Value Change {
        n1130 = event-data() -> ()  [unwired: 1 in, 5 out]
        n1131 = Or(x="Move to Position 5", y="Lower Ch. Cap.") -> (x .or. y?=w1784:bool)
        n1132 = Build Array("Move to Position 1", "Move to Position 2", "Move to Position 3", "Move to Position 4", w1784) -> (w1787:bool[])
        n1133 = Boolean Array To Number(Boolean array=w1787) -> (number=w1786:u32)
        n1134 = Logarithm Base 2(1:w1786) -> (0:w1785:dbl)
        n1135 = flat-sequence {
          tunnel: w1785 -> [w1797]
          frame #0 {
            n1136 = local read "Saved Stage Positions"() -> (w1802:dbl[][])
            n1137 = Array Subset(array=w1802, index (row)=w1797, length (row)=1 ("length"), index (col)=1 ("index"), length (col)=3 ("length")) -> (w1799:dbl[][])
            n1138 = Reshape Array(w1799, 3 ("dimension size")) -> (w1794:dbl[])
            n1139 = local write "Stage Moving"(TRUE ("Stage Moving")) -> ()
            n1140 = call "CONEX_FUNCTIONAL_GLOBAL.vi"("Axis"=enum16{"X", "Y", "Z", "XY", "XZ", "YZ", "XYZ"}."XYZ", "Position"=w1794, "Command"=T20."ABS MOVE") -> ()  [unwired: 6 in, 3 out]
          }
          frame #1 {
            n1141 = call "motor_done_moving.vi"() -> ()  [unwired: 12 in]
          }
          frame #2 {
            n1142 = local write "Stage Moving"(FALSE ("Stage Moving")) -> ()
            n1143 = call <vilib>:"Beep.vi"() -> ()  [unwired: 3 in, 9 out]
          }
        }
      }
      event "Got ADig bead": Value Change {
        n1144 = event-data() -> ()  [unwired: 1 in, 5 out]
        n1145 = property on="Move Cap. 1 (DNA Top)" class="Bool (strict)"("Val(Sgnl)"=TRUE ("Value (Signaling)")) -> ()  [unwired: 2 in, 2 out]
        n1146 = property on="Inject Bottom" class="Bool (strict)"("Val(Sgnl)"=FALSE ("Value (Signaling)")) -> ()  [unwired: 2 in, 2 out]
      }
      event "Got DNA bead": Value Change {
        n1147 = event-data() -> ()  [unwired: 1 in, 5 out]
        n1148 = property on="Cal/Data Acq. Spot" class="Bool (strict)"("Val(Sgnl)"=TRUE ("Value (Signaling)")) -> ()  [unwired: 2 in, 2 out]
        n1149 = property on="Inject Top" class="Bool (strict)"("Val(Sgnl)"=FALSE ("Value (Signaling)")) -> ()  [unwired: 2 in, 2 out]
      }
      event "Take Stepping Data": Value Change {
        n1150 = event-data() -> ()  [unwired: 1 in, 5 out]
        n1151 = local read "Save ave N"() -> (w1819:dbl)
        n1152 = flat-sequence {
          tunnel: w1819 -> [w1821]
          tunnel: [w1821] -> w1814
          tunnel: [w1823] -> w1815
          tunnel: w1814 -> [w1823]
          tunnel: [w1825] -> w1816
          tunnel: w1815 -> [w1825]
          tunnel: [w1828] -> w1817
          tunnel: w1816 -> [w1828]
          tunnel: [w1830] -> w1818
          tunnel: w1817 -> [w1830]
          tunnel: [w1832] -> w1812
          tunnel: w1818 -> [w1832]
          tunnel: w1812 -> [w1835]
          tunnel: [w1835] -> w1811
          tunnel: w1811 -> [w1836]
          tunnel: [w1836] -> w1813
          tunnel: w1813 -> [w1842]
          frame #0 {
            n1153 = property on="Save ave N" class="DigNum (strict)"("Val(Sgnl)"="Save ave factor") -> ()  [unwired: 2 in, 2 out]
          }
          frame #1 {
            n1154 = Wait (ms)(milliseconds to wait=u32 100) -> ()  [unwired: 1 out]
          }
          frame #2 {
            n1155 = local read "Offset 2 Start (MHz)"() -> (w1827:dbl)
            n1156 = property on="Saved AOD Raster Scan Parameter Sets" class="Arr (strict)"("Index Values"=u32[] [2]) -> ()  [unwired: 2 in, 2 out]
            n1157 = property on="Trap Delta (MHz)" class="DigNum (strict)"("Val(Sgnl)"=w1827) -> ()  [unwired: 2 in, 2 out]
          }
          frame #3 {
            n1158 = property on="Load parameters" class="Bool (strict)"("Val(Sgnl)"=TRUE ("Value (Signaling)")) -> ()  [unwired: 2 in, 2 out]
          }
          frame #4 {
            n1159 = Wait (ms)(milliseconds to wait=u32 100) -> ()  [unwired: 1 out]
          }
          frame #5 {
            n1160 = property on="Trap Raster Scan" class="Bool (strict)"("Val(Sgnl)"=TRUE ("Value (Signaling)")) -> ()  [unwired: 2 in, 2 out]
          }
          frame #6 {
            n1161 = Wait (ms)(milliseconds to wait=u32 1000) -> ()  [unwired: 1 out]
          }
          frame #7 {
            n1162 = while {
              stop <- w1839 stop-if-true
              n1163 = local read "Raster Scanning..."() -> (w1841:bool)
              n1164 = local read "Saving..."() -> (w1840:bool)
              n1165 = Not(x=w1840) -> (.not. x?=w1837:bool)
              n1166 = Not(x=w1841) -> (.not. x?=w1838:bool)
              n1167 = And(x=w1838, y=w1837) -> (x .and. y?=w1839:bool)
            }
          }
          frame #8 {
            n1168 = property on="Save ave N" class="DigNum (strict)"("Val(Sgnl)"=w1842) -> ()  [unwired: 2 in, 2 out]
          }
        }
      }
      event "Step Size (nm)": Value Change {
        n1169 = event-data() -> ()  [unwired: 1 in, 5 out]
        n1170 = flat-sequence {
          frame #0 {
            n1171 = property on="Saved AOD Raster Scan Parameter Sets" class="Arr (strict)"("Index Values"=u32[] [1]) -> ()  [unwired: 2 in, 2 out]
          }
          frame #1 {
            n1172 = Multiply(x="N Steps", y="Step Size (nm)") -> (x*y=w1844:dbl)
            n1173 = property on="Scan Speed AOD (nm/s) 2" class="DigNum (strict)"("Value"="Step Size (nm)") -> ()  [unwired: 2 in, 2 out]
            n1174 = property on="Step Size AOD (nm) 2" class="DigNum (strict)"("Value"="Step Size (nm)") -> ()  [unwired: 2 in, 2 out]
            n1175 = property on="Scan Range AOD (nm) 2" class="DigNum (strict)"("Value"=w1844) -> ()  [unwired: 2 in, 2 out]
          }
        }
      }
      event "Take Detection Laser\nImage": Value Change {
        n1176 = event-data() -> ()  [unwired: 1 in, 5 out]
        n1177 = flat-sequence {
          tunnel: [w1872] -> w1862
          tunnel: [w1871] -> w1855
          tunnel: [w1870] -> w1847
          tunnel: [w1875] -> w1863
          tunnel: w1862 -> [w1875]
          tunnel: [w1874] -> w1856
          tunnel: w1855 -> [w1874]
          tunnel: [w1873] -> w1848
          tunnel: w1847 -> [w1873]
          tunnel: [w1879] -> w1864
          tunnel: w1863 -> [w1879]
          tunnel: [w1878] -> w1857
          tunnel: w1856 -> [w1878]
          tunnel: [w1877] -> w1849
          tunnel: w1848 -> [w1877]
          tunnel: [w1885] -> w1865
          tunnel: w1864 -> [w1885]
          tunnel: [w1884] -> w1858
          tunnel: w1857 -> [w1884]
          tunnel: [w1883] -> w1850
          tunnel: w1849 -> [w1883]
          tunnel: [w1889] -> w1866
          tunnel: w1865 -> [w1889]
          tunnel: [w1888] -> w1859
          tunnel: w1858 -> [w1888]
          tunnel: [w1887] -> w1851
          tunnel: w1850 -> [w1887]
          tunnel: [w1893] -> w1867
          tunnel: w1866 -> [w1893]
          tunnel: [w1892] -> w1860
          tunnel: w1859 -> [w1892]
          tunnel: [w1891] -> w1852
          tunnel: w1851 -> [w1891]
          tunnel: [w1897] -> w1868
          tunnel: w1867 -> [w1897]
          tunnel: [w1896] -> w1861
          tunnel: w1860 -> [w1896]
          tunnel: [w1895] -> w1853
          tunnel: w1852 -> [w1895]
          tunnel: w1868 -> [w1903]
          tunnel: w1861 -> [w1902]
          tunnel: [w1900] -> w1854
          tunnel: w1853 -> [w1900]
          tunnel: w1854 -> [w1904]
          frame #0 {
            n1178 = local read "Green Laser ON/Interlacing"() -> (w1872:bool)
            n1179 = local read "Green laser mode"() -> (w1871:enum32{"Laser ON", "Laser OFF", "Interlace"})
            n1180 = local read "Green FB On/Off"() -> (w1870:bool)
          }
          frame #1 {
            n1181 = property on="Green FB On/Off" class="Bool (strict)"("Val(Sgnl)"=FALSE ("Value (Signaling)")) -> ()  [unwired: 2 in, 2 out]
          }
          frame #2 {
            n1182 = property on="Green Laser ON/Interlacing" class="Bool (strict)"("Val(Sgnl)"=TRUE ("Value (Signaling)")) -> ()  [unwired: 2 in, 2 out]
            n1183 = property on="Flip Green Filter" class="Bool (strict)"("Val(Sgnl)"=TRUE ("Value (Signaling)")) -> ()  [unwired: 2 in, 2 out]
            n1184 = property on="Green laser mode" class="RadioBtnsControl (strict)"("Val(Sgnl)"=enum32{"Laser ON", "Laser OFF", "Interlace"}."Laser ON" ("Value (Signaling)")) -> ()  [unwired: 2 in, 2 out]
          }
          frame #3 {
            n1185 = Wait (ms)(milliseconds to wait=u32 500) -> ()  [unwired: 1 out]
          }
          frame #4 {
            n1186 = property on="Confocal Image" class="Bool (strict)"("Val(Sgnl)"=TRUE ("Value (Signaling)")) -> ()  [unwired: 2 in, 2 out]
          }
          frame #5 {
            n1187 = Wait (ms)(milliseconds to wait=u32 2000) -> ()  [unwired: 1 out]
          }
          frame #6 {
            n1188 = while {
              stop <- w1898 stop-if-true
              n1189 = local read "Saving..."() -> (w1899:bool)
              n1190 = Not(x=w1899) -> (.not. x?=w1898:bool)
            }
          }
          frame #7 {
            n1191 = property on="Flip Green Filter" class="Bool (strict)"("Val(Sgnl)"=TRUE ("Value (Signaling)")) -> ()  [unwired: 2 in, 2 out]
            n1192 = property on="Green Laser ON/Interlacing" class="Bool (strict)"("Val(Sgnl)"=w1903) -> ()  [unwired: 2 in, 2 out]
            n1193 = property on="Green laser mode" class="RadioBtnsControl (strict)"("Val(Sgnl)"=w1902) -> ()  [unwired: 2 in, 2 out]
          }
          frame #8 {
            n1194 = property on="Green FB On/Off" class="Bool (strict)"("Val(Sgnl)"=w1904) -> ()  [unwired: 2 in, 2 out]
          }
        }
      }
      event "Stop All": Value Change {
        n1195 = event-data() -> ()  [unwired: 1 in, 5 out]
        n1196 = local read "Stop All"() -> (w1905:bool)
      }
    }
    n1197 = node-c288() -> ()  [unwired: 1 in, 1 out]
  }
  n1198 = node-c288() -> (w75:T24)  [unwired: 4 out]
  n1199 = timed-loop "Acquire Data" {
    tunnel: w16 -> [w2160]
    tunnel: w39 -> [w2159]
    tunnel: [w2190] -> w30
    tunnel: [w2184] -> w29
    timing: w163 -> [_]
    timing-out: [_] -> w162
    tunnel: w58 -> [w1988]
    stop <- "Stop All" stop-if-true
    (unwired) u32 0 ("Number of Elements")
    w1975 = "NI_ChannelName" ("name")
    n1200 = node-c288() -> ()  [unwired: 2 out]
    n1201 = First Call?() -> (First Call?: T/F=w1941:bool)
    n1202 = Or(x="Reset", y=w1941) -> (x .or. y?=w1942:bool)
    n1203 = case "Reset data stream" shown="True" w1942 {
      tunnel: w2160 -> [w2278 w2286]
      tunnel: w2159 -> [w2277 w2285]
      tunnel: [w2278 w2280] -> w2155
      tunnel: [w2277 w2279] -> w2154
      frame False {
      }
      frame True {
        w2283 = TRUE ("AI to FIFO")
        n1204 = local write "Overflow (data lost)"(FALSE ("Overflow (data lost)")) -> ()
        n1205 = call "reset FPGA DMA.vi"("error in"=w2285, "FPGA VI Reference In"=w2286) -> ("error out"=w2281:errorcluster, "FPGA VI Reference Out"=w2282:T19)
        n1206 = xnode "Read/Write Control"("FPGA VI Reference In"=w2282, "error in"=w2281, "AI to FIFO"=w2283, "APD to FIFO"=w2283) -> ("FPGA VI Reference Out"=w2280:T19, "error out"=w2279:errorcluster)
      }
    }
    n1207 = Or(x="Start AOD Scan", y="Trap Raster Scan") -> (x .or. y?=w2105:bool)
    n1208 = case "Start AOM raster scan" shown="True" w2105 {
      tunnel: w2155 -> [w3555 w3565]
      tunnel: w2154 -> [w3554 w3564]
      tunnel: [w3555 w3558] -> w2153
      tunnel: [w3554 w3557] -> w2152
      frame False {
      }
      frame True {
        n1209 = case shown="True" "Restart DMA? (AOD)" {
          tunnel: [w3603 w3605] -> w3559
          tunnel: [w3602 w3604] -> w3560
          tunnel: w3565 -> [w3603 w3607]
          tunnel: w3564 -> [w3602 w3606]
          frame False {
          }
          frame True {
            n1210 = local write "Overflow (data lost)"(FALSE ("Overflow (data lost)")) -> ()
            n1211 = call "reset FPGA DMA.vi"("error in"=w3606, "FPGA VI Reference In"=w3607) -> ("error out"=w3604:errorcluster, "FPGA VI Reference Out"=w3605:T19)
          }
        }
        n1212 = local write "Trap Raster Scan"(FALSE ("Trap Raster Scan")) -> ()
        n1213 = case shown="False" "Move MCL Also?" {
          tunnel: w3560 -> [w3568 w3597]
          tunnel: w3559 -> [w3569 w3598]
          tunnel: [w3567 w3601] -> w3558
          tunnel: [w3566 w3600] -> w3557
          frame False {
            w3570 = TRUE ("AI to FIFO")
